vi "Select Opamp.vi"(8 "error in (no error)":errorcluster) -> (0 "error out":errorcluster, 3 "Opamp Type":T1)   [LabVIEW 2018]
uses:
  type defs/OpAmp Amplifiers.ctl
  type defs/AmplifierTypes.ctl
panel:
  in  "Cancel Button":bool
  in  "Amplifier Type":T2 caption="Trans Type"
  in  "Opamp Type":T1 caption="OpAmp"
  in  "Non INV":bool
  in  "INV":bool
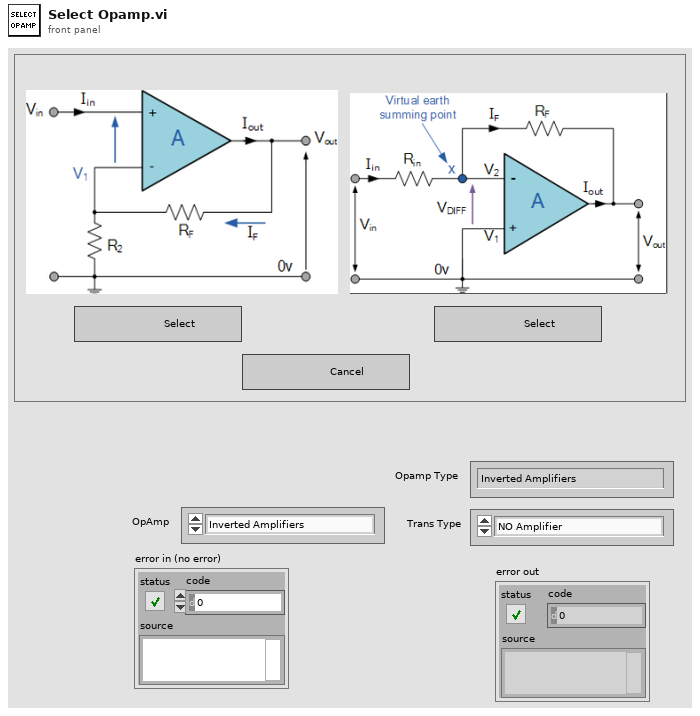
[diagram p1: front panel]
types:
  T1 = typedef "OpAmp Amplifiers.ctl" = enum8{"Inverted Amplifiers", "non-Inverted Amplifiers", "NO Amplifier"}
  T2 = typedef "AmplifierTypes.ctl" = enum8{"NO Amplifier", "EC", "BC", "CC"}
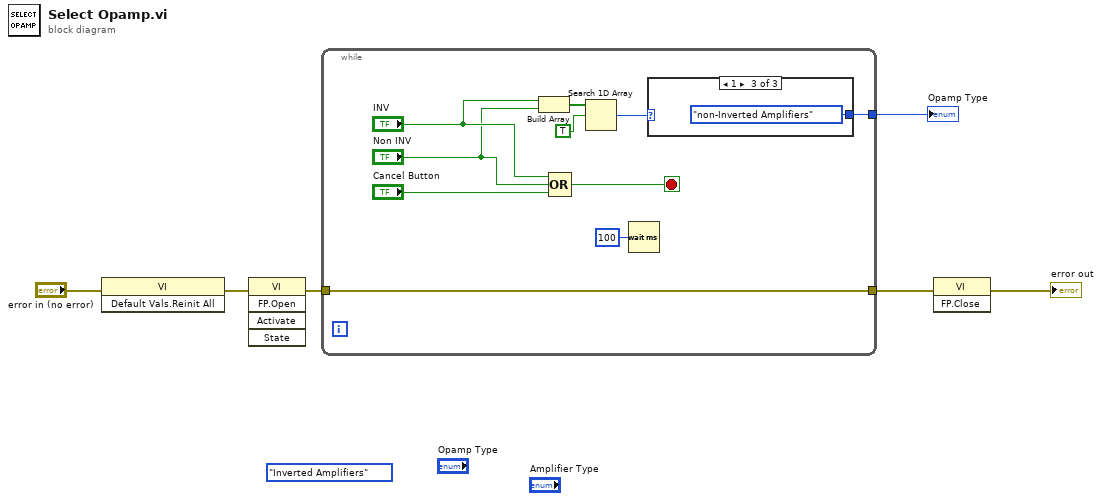
[diagram p0: block diagram]
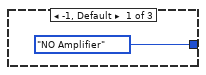
[diagram p2: hidden frame]
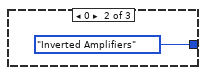
[diagram p3: hidden frame]
diagram:
  (unwired) OpAmp_Amplifiers."Inverted Amplifiers" ("Opamp Type")
  n1 = invoke class="VI" method="Default Vals.Reinit All"(error in="error in (no error)") -> (error out=w3:errorcluster)  [unwired: 2 in, 2 out]
  n2 = invoke class="VI" method="FP.Open"(error in=w3) -> (error out=w6:errorcluster)  [unwired: 4 in, 4 out]
  n3 = while {
    tunnel: w6 -> [w9]
    tunnel: [w9] -> w1
    tunnel: [w7] -> w5
    stop <- w16 stop-if-true
    n4 = Build Array("INV", "Non INV") -> (w12:bool[])
    n5 = Compound Arithmetic op=OR("INV", "Non INV", "Cancel Button") -> (w16:bool)
    n6 = Search 1D Array(1D array=w12, element=TRUE) -> (index of element=w10:i32)  [unwired: 1 in]
    n7 = Wait (ms)(milliseconds to wait=u32 100) -> ()  [unwired: 1 out]
    n8 = case shown="1" w10 {
      tunnel: [OpAmp_Amplifiers."NO Amplifier" ("Opamp Type") OpAmp_Amplifiers."Inverted Amplifiers" ("Opamp Type") OpAmp_Amplifiers."non-Inverted Amplifiers" ("Opamp Type")] -> w7
      frame -1, Default {
      }
      frame 0 {
      }
      frame 1 {
      }
    }
  }
  "Opamp Type" <- w5
  n9 = invoke class="VI" method="FP.Close"(error in=w1) -> (error out=→"error out":errorcluster)  [unwired: 2 in, 2 out]
